vi "Detect Network Devices.vi"(4 "Remote Timeout":u32=300000 caption="Remote Timeout (300,000 ms)", 7 "Local Subnet Only":bool caption="Local Subnet Only (F)", 8 "error in":errorcluster caption="Error in", 9 "Device Class String":string[](array[string]), 10 "Device Class":T2, 11 "Session in (localhost)":refnum<k21>="localhost") -> (0 "Error out":errorcluster, 1 "Devices Skipped":T1[](array[typedef]) {"Product ID" format="%.0x"}, 2 "Devices Found":T1[](array[typedef]) {"Product ID" format="%.0x"}, 3 "Session out":refnum<k21>)   [LabVIEW 2015, in "SMI.lvlib" / "Device.lvclass"]
uses:
  Device.lvclass
  Controls/DeviceClassSelection.ctl
  Controls/NetworkDeviceInformation.ctl
  <vilib>/nisyscfg/Filter Mode.ctl
  <vilib>/nisyscfg/Close (Resources).vi
  <vilib>/regexp/Match Regular Expression.xnode
  <vilib>/nisyscfg/Close (Filter).vi
  <vilib>/nisyscfg/nisyscfg.lvlib
  <resource>/objmgr/niflexriosae.rc
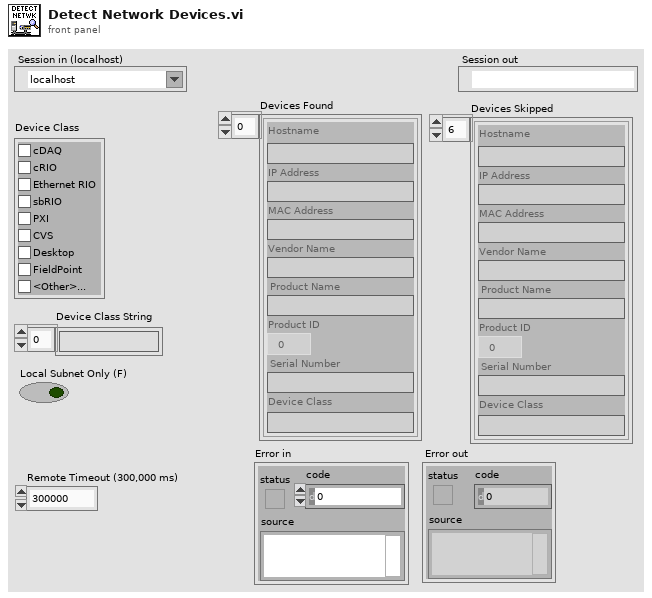
[diagram p1: front panel]
types:
  T1 = typedef "SMI.lvlib/Device.lvclass/NetworkDeviceInformation.ctl" = cluster{"Hostname":string, "IP Address":string, "MAC Address":string, "Vendor Name":string, "Product Name":string, "Product ID":u16, "Serial Number":string, "Device Class":string}
  T2 = typedef "SMI.lvlib/Device.lvclass/DeviceClassSelection.ctl" = cluster{"cDAQ":bool, "cRIO":bool, "Ethernet RIO":bool, "sbRIO":bool, "PXI":bool, "CVS":bool, "Desktop":bool, "FieldPoint":bool, "<Other>...":bool}
  T3 = typedef "nisyscfg.lvlib/Filter Mode.ctl" = i32
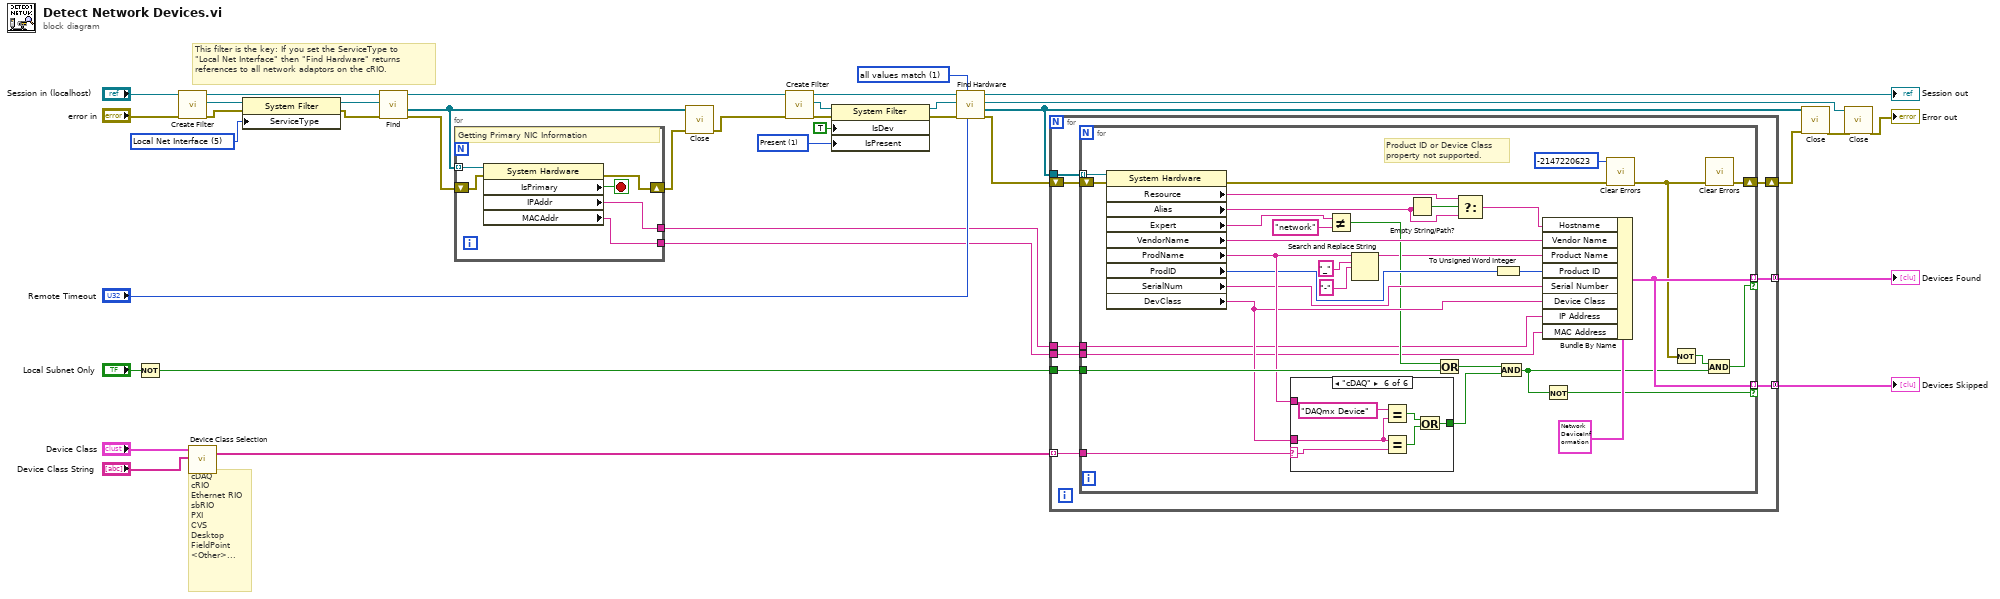
[diagram p0: block diagram]
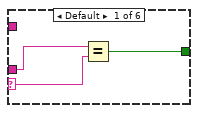
[diagram p2: hidden frame]
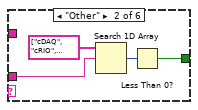
[diagram p3: hidden frame]
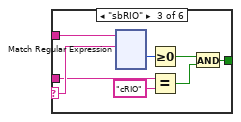
[diagram p4: hidden frame]
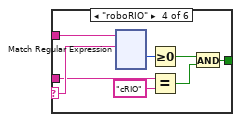
[diagram p5: hidden frame]
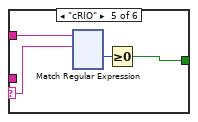
[diagram p6: hidden frame]
diagram:
  w2 = 1 items=["Initializing"=-2, "Unknown"=-1, "Not Present"=0, "Present"=1] ("Devices & Chassis:Is Present")
  w13 = u32 5 items=["NI Network Resource", "NI Real-Time", "NI System Configuration", "NI Web Interface", "Local System", "Local Net Interface", "Local Time Keeper", "Local Time Reference", "LXI Instrument"] ("Service Type")
  w29 = T3 1 items=["all values match"=1, "any value matches"=2, "values do not match"=3, "all properties exist"=4] ("filter mode (all values match)")
  # "This filter is the key: If you set the ServiceType to\n\"Local Net Interface\" then \"Find Hardware\" returns\nreferences to all network adaptors on the cRIO."
  # "cDAQ\ncRIO\nEthernet RIO\nsbRIO\nPXI\nCVS\nDesktop\nFieldPoint\n<Other>..."
  n1 = Not(x="Local Subnet Only") -> (.not. x?=w35:bool)
  n2 = call <vilib>:"Create Filter.vi"("error in (no error)"="error in", "Session in"="Session in (localhost)") -> ("error out"=w16:errorcluster, "Filter out"=w12:refnum<k20>, "Session out"=w11:refnum<k21>)  [unwired: 7 in]
  n3 = call "Device Class Selection.vi"("Device Class Strings"="Device Class String", "Device Classes"="Device Class") -> ("Device Class"=w18:string[])  [unwired: 3 in]
  n4 = property class="System Filter"(reference=w12, error in=w16, "ServiceType"=w13) -> (reference out=w14:refnum<k20>, error out=w15:errorcluster)
  n5 = call-poly <vilib>:"Find.vi"("error in (no error)"=w15, "Filter in"=w14, "Session in"=w11) -> ("error out"=w17:errorcluster, "Resources out"=w5:refnum<k20>[], "Session out"=w8:refnum<k21>)  [unwired: 5 in, 1 out]
  n6 = for {
    tunnel: w5 -> [w43] mode=indexing
    shift-right: [w42] -> w4
    shift-left: w17 -> [w44]
    tunnel: [w40] -> w7
    tunnel: [w39] -> w6
    stop <- w41 stop-if-true
    # "Getting Primary NIC Information"
    n7 = property class="System Hardware"(reference=w43, error in=w44) -> (error out=w42:errorcluster, "IsPrimary"=w41:bool, "IPAddr"=w40:string, "MACAddr"=w39:string)  [unwired: 1 out]
  }
  n8 = call-poly <vilib>:"Close.vi"("error in (no error)"=w4, "Resources in"=w5) -> ("error out"=w3:errorcluster)  [unwired: 9 in]
  n9 = call <vilib>:"Create Filter.vi"("error in (no error)"=w3, "Session in"=w8) -> ("error out"=w34:errorcluster, "Filter out"=w33:refnum<k20>, "Session out"=w32:refnum<k21>)  [unwired: 7 in]
  n10 = property class="System Filter"(reference=w33, error in=w34, "IsDev"=TRUE ("Is Chassis"), "IsPresent"=w2) -> (reference out=w30:refnum<k20>, error out=w31:errorcluster)
  n11 = call <vilib>:"Find Hardware.vi"("Remote Timeout (300,000 ms)"="Remote Timeout", "Filter Mode (all values match)"=w29, "error in (no error)"=w31, "Filter in"=w30, "Session in"=w32) -> ("error out"=w28:errorcluster, "Resources out"=w27:refnum<k20>[], "Filter out"=w25:refnum<k20>, "Session out"=→"Session out":refnum<k21>)  [unwired: 3 out]
  n12 = for {
    tunnel: w35 -> [w53]
    tunnel: w27 -> [w51]
    tunnel: [w49] -> w22 mode=concatenating
    tunnel: w18 -> [w48] mode=indexing
    shift-right: [w50] -> w24
    shift-left: w28 -> [w52]
    tunnel: w7 -> [w47]
    tunnel: w6 -> [w46]
    tunnel: [w45] -> w1 mode=concatenating
    n13 = for {
      tunnel: w51 -> [w87] mode=indexing
      shift-right: [w80] -> w50
      shift-left: w52 -> [w86]
      tunnel: w53 -> [w85]
      tunnel: [w58] -> w49 mode=indexing if=w55
      tunnel: w48 -> [w74]
      tunnel: w47 -> [w60]
      tunnel: w46 -> [w61]
      tunnel: [w58] -> w45 mode=indexing if=w57
      # "Product ID or Device Class\nproperty not supported."
      n14 = property class="System Hardware"(reference=w87, error in=w86) -> (error out=w79:errorcluster, "Resource"=w83:string, "Alias"=w84:string, "Expert"=w82:string, "VendorName"=w81:string, "ProdName"=w78:string, "ProdID"=w75:u32, "SerialNum"=w76:string, "DevClass"=w77:string)  [unwired: 1 out]
      n15 = case shown="\"cDAQ\"" w74 {
        selector: w74 -> [w90 _ w101 w223 w341 w459]
        tunnel: w77 -> [w89 w93 w100 w222 _ w458]
        tunnel: w78 -> [_ _ w102 w224 w342 _]
        tunnel: [w88 w91 w96 w218 w339 w460] -> w68
        frame Default {
          n16 = Equal?(x=w89, y=w90) -> (x = y?=w88:bool)
        }
        frame "Other" {
          n17 = Search 1D Array(1D array=string[] ["cDAQ", "cRIO", "Ethernet RIO", "sbRIO", "PXI", "CVS", "Desktop", "FieldPoint"], element=w93) -> (index of element=w92:i32)  [unwired: 1 in]
          n18 = Less Than 0?(x=w92) -> (x < 0?=w91:bool)
        }
        frame "sbRIO" {
          n19 = xnode "Match Regular Expression"("input string"=w102, "regular expression"=w101) -> ("offset past match"=w99:i32)  [unwired: 4 in, 4 out]
          n20 = Greater Or Equal To 0?(x=w99) -> (x >= 0?=w97:bool)
          n21 = Equal?(x=w100, y="cRIO") -> (x = y?=w98:bool)
          n22 = And(x=w97, y=w98) -> (x .and. y?=w96:bool)
        }
        frame "roboRIO" {
          n23 = xnode "Match Regular Expression"("input string"=w224, "regular expression"=w223) -> ("offset past match"=w221:i32)  [unwired: 4 in, 4 out]
          n24 = Greater Or Equal To 0?(x=w221) -> (x >= 0?=w219:bool)
          n25 = Equal?(x=w222, y="cRIO") -> (x = y?=w220:bool)
          n26 = And(x=w219, y=w220) -> (x .and. y?=w218:bool)
        }
        frame "cRIO" {
          n27 = xnode "Match Regular Expression"("input string"=w342, "regular expression"=w341) -> ("offset past match"=w340:i32)  [unwired: 4 in, 4 out]
          n28 = Greater Or Equal To 0?(x=w340) -> (x >= 0?=w339:bool)
        }
        frame "cDAQ" {
          n29 = Equal?(x="DAQmx Device", y=w458) -> (x = y?=w462:bool)
          n30 = Equal?(x=w458, y=w459) -> (x = y?=w461:bool)
          n31 = Or(x=w462, y=w461) -> (x .or. y?=w460:bool)
        }
      }
      n32 = Not Equal?(x=w82, y="network") -> (x != y?=w71:bool)
      n33 = Search and Replace String(input string=w78, search string="_", replace string="-" ("replace string (\"\")")) -> (result string=w64:string)  [unwired: 5 in, 3 out]
      n34 = Empty String/Path?(string/path=w84) -> (empty?=w73:bool)
      n35 = Or(x=w71, y=w85) -> (x .or. y?=w67:bool)
      n36 = Select(t=w83, s=w73, f=w84) -> (s? t:f=w59:string)
      n37 = To Unsigned Word Integer(number=w75) -> (unsigned 16bit integer=w63:u16)
      n38 = And(x=w67, y=w68) -> (x .and. y?=w56:bool)
      n39 = Bundle By Name(cluster=T1 {"Hostname"="cRIO-9014-Test", "IP Address"="", "MAC Address"="", "Vendor Name"="National Instruments", "Product Name"="", "Product ID"=29071, "Serial Number"="00E86EAB", "Device Class"=""} ("Device Information"), "Hostname"=w59, "Vendor Name"=w81, "Product Name"=w64, "Product ID"=w63, "Serial Number"=w76, "Device Class"=w77, "IP Address"=w60, "MAC Address"=w61) -> (w58:T1)
      n40 = Not(x=w56) -> (.not. x?=w55:bool)
      n41 = call <vilib>:"Clear Errors.vi"("error in (no error)"=w79, "specific error code to clear (0: all)"=-2147220623) -> ("error out"=w54:errorcluster)  [unwired: 4 in, 1 out]
      n42 = Not(x=w54) -> (.not. x?=w69:bool)
      n43 = call <vilib>:"Clear Errors.vi"("error in (no error)"=w54) -> ("error out"=w80:errorcluster)  [unwired: 5 in, 1 out]
      n44 = And(x=w69, y=w56) -> (x .and. y?=w57:bool)
    }
  }
  "Devices Found" <- w1
  "Devices Skipped" <- w22
  n45 = call-poly <vilib>:"Close.vi"("error in (no error)"=w24, "Resources in"=w27) -> ("error out"=w23:errorcluster)  [unwired: 9 in]
  n46 = call-poly <vilib>:"Close.vi"("error in (no error)"=w23, "Filter in"=w25) -> ("error out"=→"Error out":errorcluster)  [unwired: 9 in]
